vi "DLG - Ask Duration sec.vi"() -> (13 "Segment Length (sec)":string)   [LabVIEW 2020, in "SPWB.lvclass"]
uses:
  SPWB.lvclass
panel:
  in  "OK Button":bool
  in  "Segment Length (sec)":dbl min=0.0 max=100.0 step=0.1
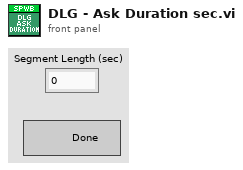
[diagram p1: front panel]
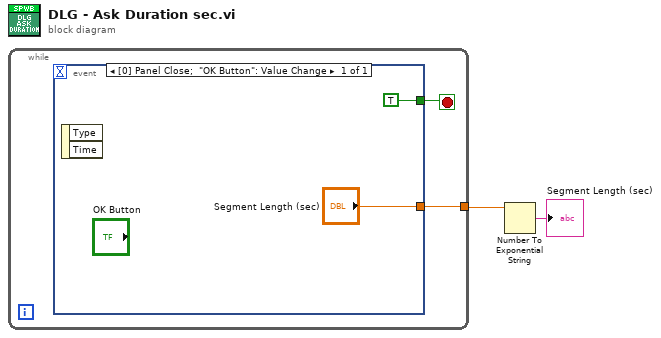
[diagram p0: block diagram]
diagram:
  n1 = while {
    tunnel: [w3] -> w2
    stop <- w4 stop-if-true
    n2 = event shown="[0] Panel Close;  \"OK Button\": Value Change" {
      selector: _ -> [_]
      dyn-events: _ -> [_]
      timeout: _ -> [_]
      tunnel: [TRUE] -> w4
      tunnel: ["Segment Length (sec)"] -> w3
      event Panel Close; "OK Button": Value Change {
        n3 = event-data() -> ()  [unwired: 1 in, 2 out]
      }
    }
  }
  n4 = Number To Exponential String(number=w2) -> (E-format string=→"Segment Length (sec)":string)  [unwired: 3 in]
